vi "Encoder.vi"() -> ()   [LabVIEW 2013]
uses:
  <vilib>/Rock Robotics/SystemInterfaces/DIO/FPGA_DIOChannel.ctl
  <vilib>/Rock Robotics/SystemInterfaces/DIO/FPGA_DIOPWMChannel.ctl
  <vilib>/Rock Robotics/WPI/MotorControl/WPI_MotorControlOpen Jaguar.vi
panel:
  in  "Output":dbl(slide) scale=-1.0..1.0
  in  "stop":bool
  out "Waveform Chart":i16[](graph)
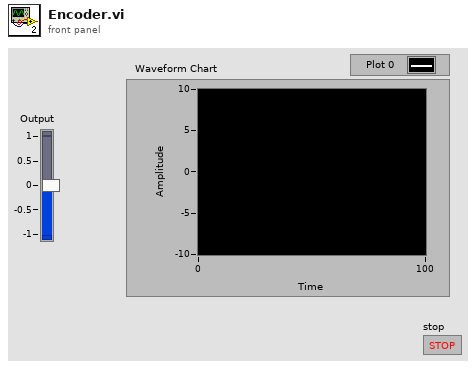
[diagram p1: front panel]
types:
  T1 = typedef "FPGA_DIOPWMChannel.ctl" = enum8{"PWM 1", "PWM 2", "PWM 3", "PWM 4", "PWM 5", "PWM 6", "PWM 7", "PWM 8", "PWM 9", "PWM 10", "Invalid"}
  T2 = typedef "FPGA_DIOChannel.ctl" = enum8{"DIO 1", "DIO 2", "DIO 3", "DIO 4", "DIO 5", "DIO 6", "DIO 7", "DIO 8", "DIO 9", "DIO 10", "DIO 11", "DIO 12", "DIO 13", "DIO 14", "Invalid"}
  T3 = typedef "WPI_MotorControlDeviceRef.ctl" = cluster{"DeviceStatus":errorcluster, "Type":enum16{"PWM", "CAN"}, "PWM":cluster{"Digital Module":T4, "PWM Channel":T1, "DeadBand":T5}, "CAN":cluster{"Device Number":u8, "Control Mode":T6, "Semaphore":T7, "Max Vout":dbl}, "Invert":bool, "TransformRef":T8, "InvTransformRef":T8}
  T4 = typedef "FPGA_TypedefDigitalModule.ctl" = enum16{"Digital Module 1", "Digital Module 2"}
  T5 = typedef "WPI_PWMDeadband.ctl" = cluster{"Name":string, "maxPositivePwm":i32, "minPositivePwm":i32, "centerPwm":i32, "maxNegativePwm":i32, "minNegativePwm":i32, "angularRange":u16}
  T6 = typedef "WPI_CANJaguar_ControlMode.ctl" = enum8{"Percent VBus", "Current", "Speed", "Position", "Voltage"}
  T7 = typedef "Semaphore RefNum" = refnum<k1>
  T8 = typedef "WPI_PWMTransform_ConPane.ctl" = refnum<vi>
  T9 = typedef "WPI_DigitalInputDevRef.ctl" = cluster{"DevStatus":errorcluster, "DIO Channel":T2, "Digital Module":T4}
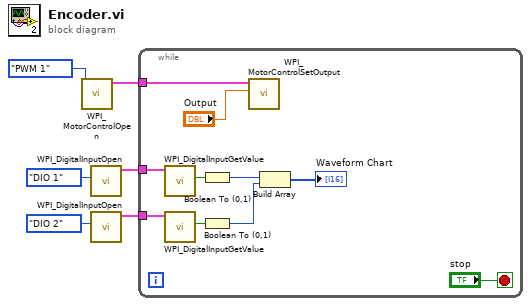
[diagram p0: block diagram]
diagram:
  n1 = call-poly <vilib>:"WPI_MotorControlOpen.vi"("PWM Channel"=FPGA_DIOPWMChannel."PWM 1") -> ("MotorControlDeviceRef"=w2:T3)  [unwired: 9 in, 1 out]
  n2 = call <vilib>:"WPI_DigitalInputOpen.vi"("DIO Channel"=FPGA_DIOChannel."DIO 1") -> ("DigitalInputDevRef"=w6:T9)  [unwired: 9 in, 1 out]
  n3 = call <vilib>:"WPI_DigitalInputOpen.vi"("DIO Channel"=FPGA_DIOChannel."DIO 2") -> ("DigitalInputDevRef"=w5:T9)  [unwired: 9 in, 1 out]
  n4 = while {
    tunnel: w6 -> [w16]
    tunnel: w5 -> [w15]
    tunnel: w2 -> [w8]
    stop <- "stop" stop-if-true
    n5 = call <vilib>:"WPI_DigitalInputGetValue.vi"("DigitalInputDevRef"=w16) -> ("Value"=w14:bool)  [unwired: 8 in, 2 out]
    n6 = call <vilib>:"WPI_DigitalInputGetValue.vi"("DigitalInputDevRef"=w15) -> ("Value"=w13:bool)  [unwired: 8 in, 2 out]
    n7 = Boolean To (0,1)(Boolean=w14) -> (0, 1=w12:i16)
    n8 = Boolean To (0,1)(Boolean=w13) -> (0, 1=w11:i16)
    n9 = call <vilib>:"WPI_MotorControlSetOutput.vi"("Output"="Output", "MotorControlDevRef"=w8) -> ()  [unwired: 7 in, 3 out]
    n10 = Build Array(w12, w11) -> (→"Waveform Chart":i16[])
  }
